vi "Average data.vi"(9 "Numeric":i32, 10 "Array":dbl[](array[numeric]), 11 "file path (dialog if empty)":path) -> (1 "XY Graph":cluster{"Y":dbl[], "Y":dbl[]}[](graph))   [LabVIEW 2011]
uses:
  <vilib>/Utility/file.llb/Read From Spreadsheet File (DBL).vi
  <vilib>/Analysis/NI_AALBase.lvlib
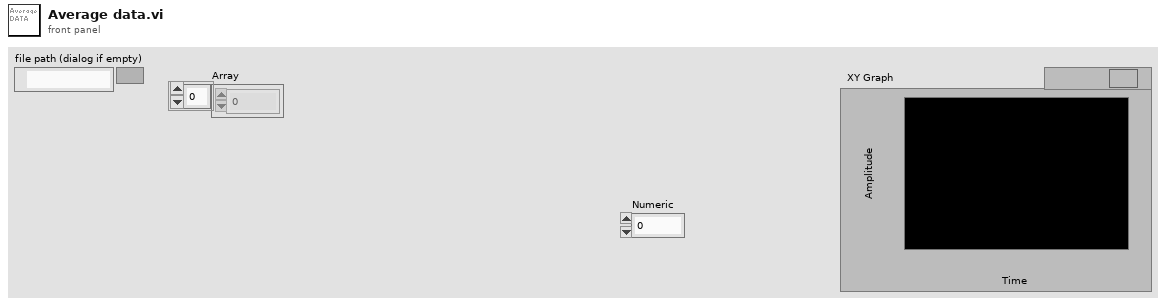
[diagram p1: front panel]
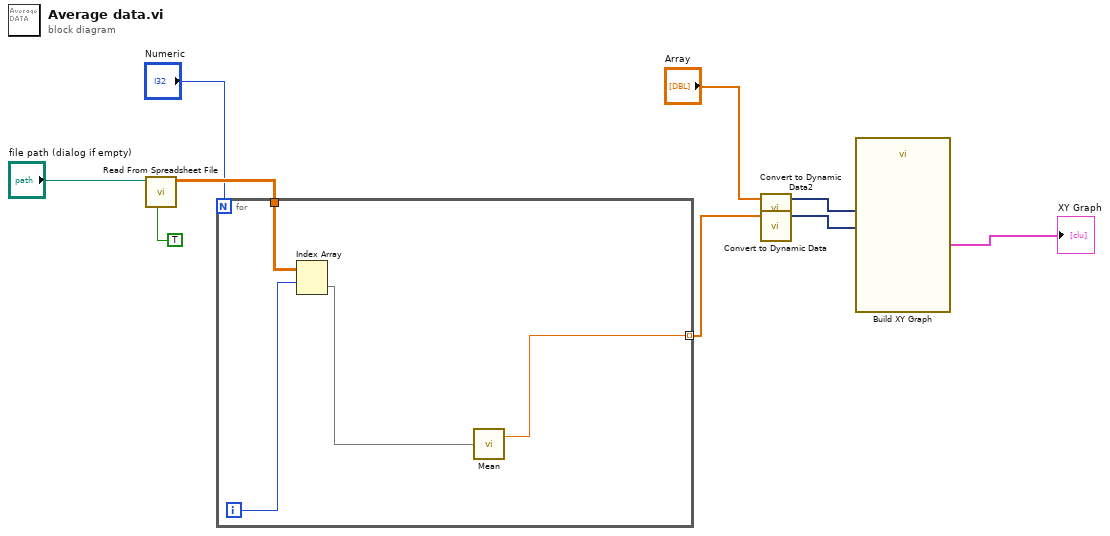
[diagram p0: block diagram]
diagram:
  n1 = call-poly <vilib>:"Read From Spreadsheet File.vi"("transpose (no:F)"=TRUE, "file path (dialog if empty)"="file path (dialog if empty)") -> ("all rows"=w8:dbl[][])  [unwired: 5 in, 4 out]
  n2 = for {
    N: "Numeric" -> [_]
    tunnel: w8 -> [w13]
    tunnel: [w11] -> w3 mode=indexing
    i -> [w12]
    n3 = Index Array(array=w13, index (row)=w12) -> (element=w10:dbl[])  [unwired: 1 in]
    n4 = call <vilib>:"Mean.vi"("X"=w10) -> ("mean"=w11:dbl)  [unwired: 1 out]
  }
  n5 = call "Convert to Dynamic Data2"("Array"="Array") -> ("Dynamic Data Type"=w4:dynamicdata)  [unwired: 3 in]
  n6 = call "Convert to Dynamic Data"("Array"=w3) -> ("Dynamic Data Type"=w5:dynamicdata)  [unwired: 3 in]
  n7 = call "Build XY Graph"("Y Input"=w5, "X Input"=w4) -> ("XY Graph"=→"XY Graph":cluster{"Y":dbl[], "Y":dbl[]}[])  [unwired: 3 in, 6 out]
